vi "Machine.vi"   [LabVIEW 2011]
doc: "使用该模板构建标准状态机设计模式。各状态执行代码并决定转移状态。将该设计模式与根据用户动作响应而执行代码的用户界面事件处理器模式相比较。同时将该设计模式与队列消息处理模式（各消息处理代码可排队0个或多个新消息）。"
uses:
  MachineState.ctl
  F1State.ctl
  API/API DYM.lvlib
types:
  T1 = typedef "MachineState.ctl" = enum16{"Initialize", "一号平台分拣运输", "二号平台运输物料", "三号平台气动机械手运输物料", "三号平台运输机构运输物料", "Stop"}
  T2 = typedef "F1State.ctl" = enum16{"Initialize", "Stop", "推送物料", "推料气缸复位", "物件到位检测-光电漫射", "物体属性检测-电涡流", "分拣物体", "不分拣物体", "物件到位检测-电容式接近开关", "气缸机构运动", "气缸机构复位"}
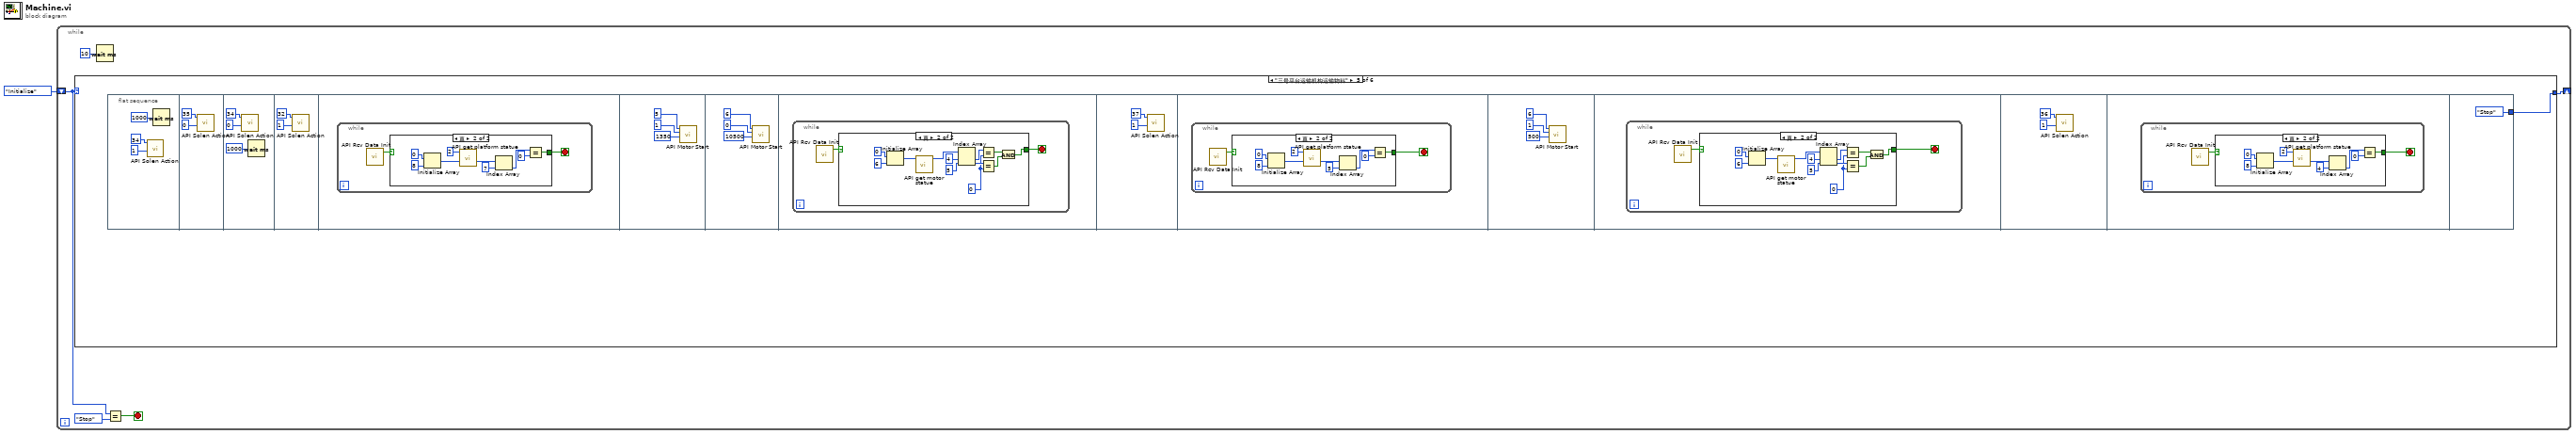
[diagram p0: block diagram]
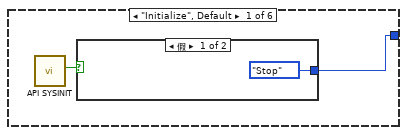
[diagram p2: hidden frame]
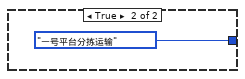
[diagram p3: hidden frame]
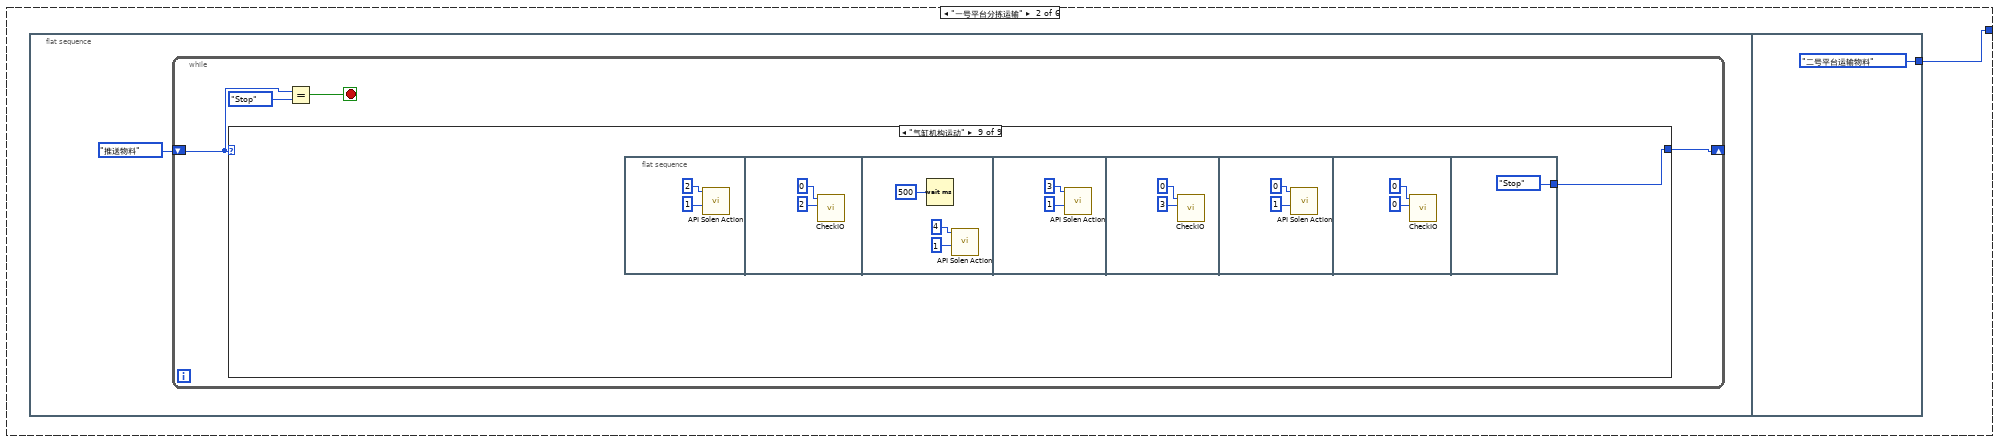
[diagram p4: hidden frame]
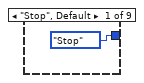
[diagram p5: hidden frame]
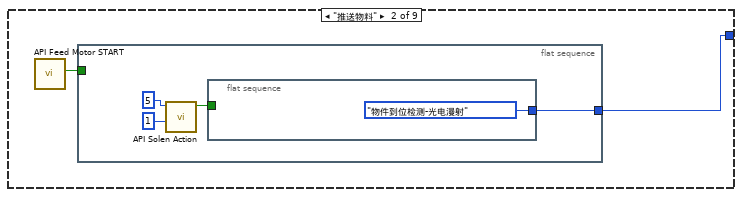
[diagram p6: hidden frame]
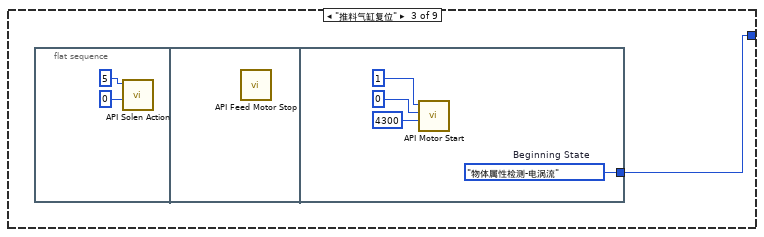
[diagram p7: hidden frame]
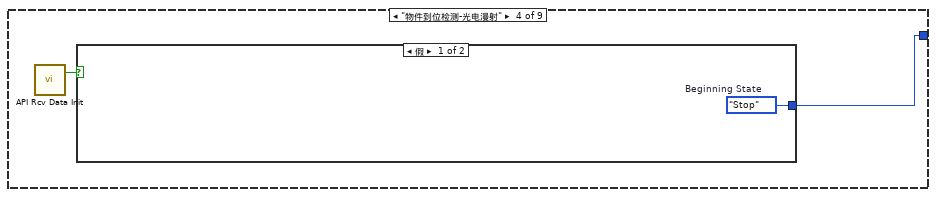
[diagram p8: hidden frame]
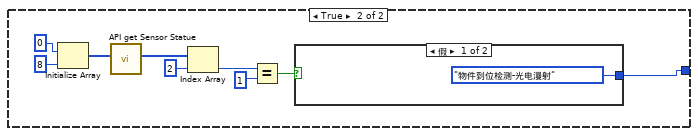
[diagram p9: hidden frame]
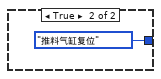
[diagram p10: hidden frame]
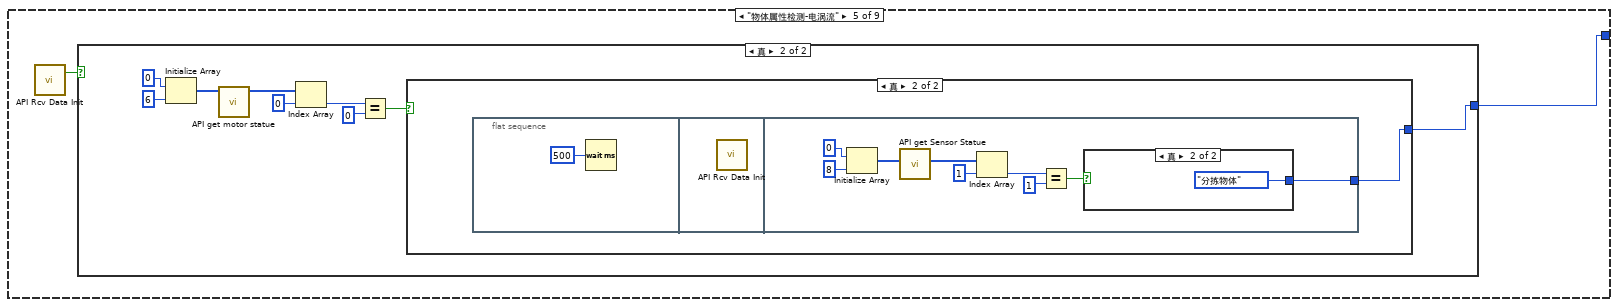
[diagram p11: hidden frame]
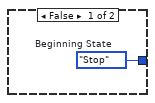
[diagram p12: hidden frame]
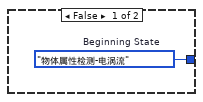
[diagram p13: hidden frame]
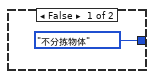
[diagram p14: hidden frame]
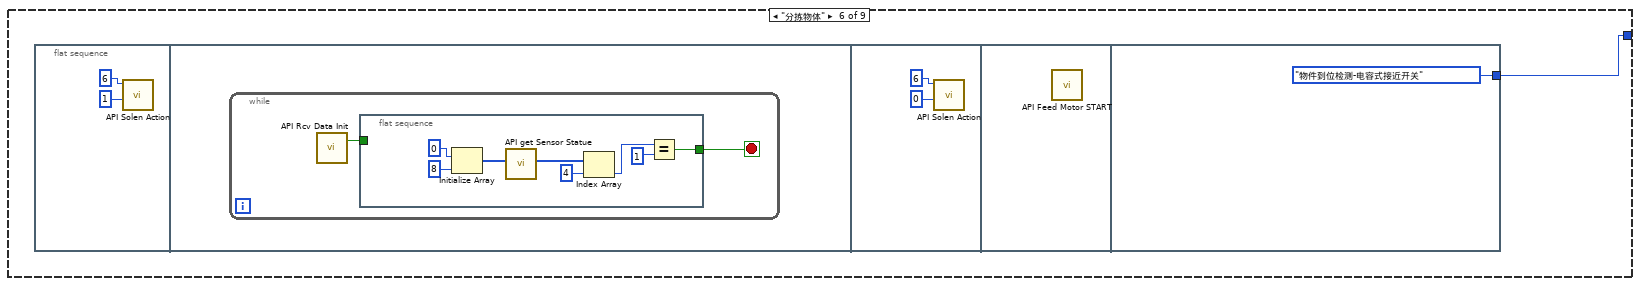
[diagram p15: hidden frame]
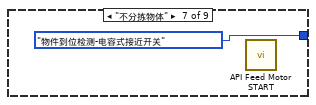
[diagram p16: hidden frame]
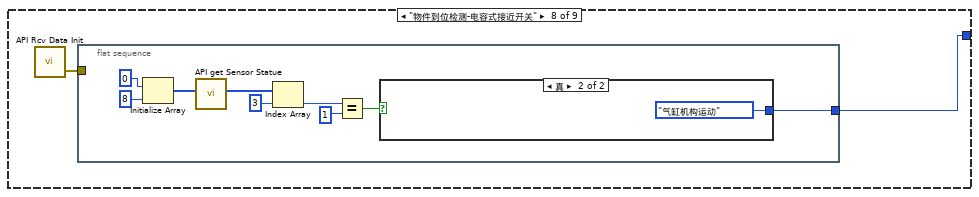
[diagram p17: hidden frame]
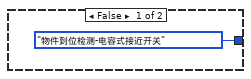
[diagram p18: hidden frame]
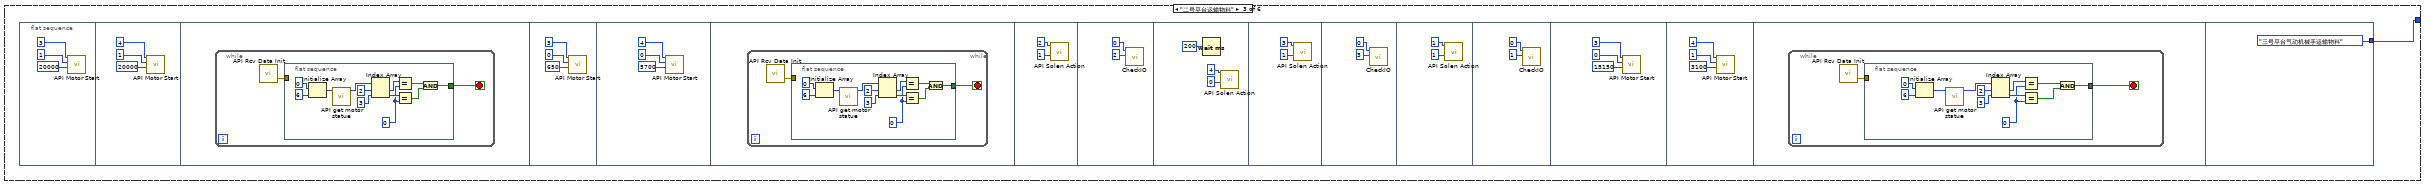
[diagram p19: hidden frame]
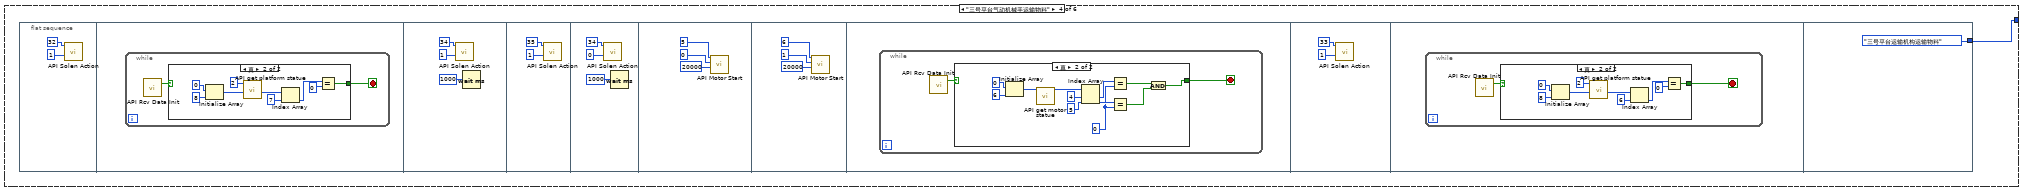
[diagram p20: hidden frame]
diagram:
  n1 = while {
    shift-right: [w2] -> _
    shift-left: MachineState."Initialize" ("Beginning State") -> [w4]
    stop <- w6 stop-if-true
    n2 = case shown="\"三号平台运输机构运输物料\"" w4 {
      tunnel: [w7 w11 w120 w197 w256 MachineState."Stop" ("Beginning State")] -> w2
      frame "Initialize", Default {
        n3 = call "API SYSINIT.vi"() -> ("SYSINIT return value"=w8:bool)  [unwired: 11 in]
        n4 = case shown="假" w8 {
          tunnel: [MachineState."Stop" ("Beginning State") MachineState."一号平台分拣运输" ("Beginning State")] -> w7
          frame False {
          }
          frame True {
          }
        }
      }
      frame "一号平台分拣运输" {
        n5 = flat-sequence {
          tunnel: [MachineState."二号平台运输物料" ("Beginning State")] -> w11
          frame #0 {
            n6 = while {
              shift-right: [w13] -> _
              shift-left: F1State."推送物料" ("Beginning State") -> [w14]
              stop <- w16 stop-if-true
              n7 = case shown="\"气缸机构运动\"" w14 {
                tunnel: [F1State."Stop" ("Beginning State") w19 w25 w32 w46 w72 F1State."物件到位检测-电容式接近开关" ("Beginning State") w89 w102] -> w13
                frame "Stop", Default {
                }
                frame "推送物料" {
                  n8 = call "API Feed Motor START.vi"() -> ("feedmotorstart return value"=w18:bool)  [unwired: 11 in]
                  n9 = flat-sequence {
                    tunnel: [w20] -> w19
                    tunnel: w18 -> [_]
                    frame #0 {
                      n10 = call "API Solen Action.vi"("statue"=1, "solenNum"=5) -> ("solenaction return value"=w21:bool)  [unwired: 9 in]
                      n11 = flat-sequence {
                        tunnel: w21 -> [_]
                        tunnel: [F1State."物件到位检测-光电漫射" ("Beginning State")] -> w20
                        frame #0 {
                        }
                      }
                    }
                  }
                }
                frame "推料气缸复位" {
                  n12 = flat-sequence {
                    tunnel: [w28] -> w25
                    frame #0 {
                      n13 = call "API Solen Action.vi"("statue"=0, "solenNum"=5) -> ()  [unwired: 9 in, 1 out]
                    }
                    frame #1 {
                      n14 = call "API Feed Motor Stop.vi"() -> ()  [unwired: 11 in, 1 out]
                    }
                    frame #2 {
                      w28 = F1State."物体属性检测-电涡流"  # Beginning State
                      n15 = call "API Motor Start.vi"("stepNum"=4300, "direction"=0, "motorNum"=1) -> ()  [unwired: 8 in, 1 out]
                    }
                  }
                }
                frame "物件到位检测-光电漫射" {
                  n16 = call "API Rcv Data Init.vi"() -> ("RTV"=w33:bool)  [unwired: 2 in, 1 out]
                  n17 = case shown="假" w33 {
                    tunnel: [w34 w35] -> w32
                    frame False {
                      w34 = F1State."Stop"  # Beginning State
                    }
                    frame True {
                      n18 = Initialize Array(0 ("元素"), 8 ("维数大小")) -> (w41:i32[])
                      n19 = call "API get Sensor Statue.vi"("array input"=w41) -> ("array output"=w40:i32[])  [unwired: 9 in, 1 out]
                      n20 = Index Array(array=w40, index=2 ("索引")) -> (element=w38:i32)
                      n21 = Equal?(x=w38, y=1) -> (x = y?=w36:bool)
                      n22 = case shown="假" w36 {
                        tunnel: [F1State."物件到位检测-光电漫射" ("Beginning State") F1State."推料气缸复位" ("Beginning State")] -> w35
                        frame False {
                        }
                        frame True {
                        }
                      }
                    }
                  }
                }
                frame "物体属性检测-电涡流" {
                  n23 = call "API Rcv Data Init.vi"() -> ("RTV"=w47:bool)  [unwired: 2 in, 1 out]
                  n24 = case shown="真" w47 {
                    tunnel: [w48 w49] -> w46
                    frame False {
                      w48 = F1State."Stop"  # Beginning State
                    }
                    frame True {
                      n25 = Initialize Array(0 ("元素"), 6 ("维数大小")) -> (w55:i32[])
                      n26 = call "API get motor statue.vi"("motor statue array input"=w55) -> ("motor statue array output"=w54:i32[])  [unwired: 9 in, 1 out]
                      n27 = Index Array(array=w54, index=0 ("索引")) -> (element=w52:i32)
                      n28 = Equal?(x=w52, y=0) -> (x = y?=w50:bool)
                      n29 = case shown="真" w50 {
                        tunnel: [w58 w59] -> w49
                        frame False {
                          w58 = F1State."物体属性检测-电涡流"  # Beginning State
                        }
                        frame True {
                          n30 = flat-sequence {
                            tunnel: [w61] -> w59
                            frame #0 {
                              n31 = Wait (ms)(milliseconds to wait=u32 500) -> ()  [unwired: 1 out]
                            }
                            frame #1 {
                              n32 = call "API Rcv Data Init.vi"() -> ()  [unwired: 2 in, 2 out]
                            }
                            frame #2 {
                              n33 = Initialize Array(0 ("元素"), 8 ("维数大小")) -> (w67:i32[])
                              n34 = call "API get Sensor Statue.vi"("array input"=w67) -> ("array output"=w66:i32[])  [unwired: 9 in, 1 out]
                              n35 = Index Array(array=w66, index=1 ("索引")) -> (element=w63:i32)
                              n36 = Equal?(x=w63, y=1) -> (x = y?=w62:bool)
                              n37 = case shown="真" w62 {
                                tunnel: [F1State."不分拣物体" ("Beginning State") F1State."分拣物体" ("Beginning State")] -> w61
                                frame False {
                                }
                                frame True {
                                }
                              }
                            }
                          }
                        }
                      }
                    }
                  }
                }
                frame "分拣物体" {
                  n38 = flat-sequence {
                    tunnel: [F1State."物件到位检测-电容式接近开关" ("Beginning State")] -> w72
                    frame #0 {
                      n39 = call "API Solen Action.vi"("statue"=1, "solenNum"=6) -> ()  [unwired: 9 in, 1 out]
                    }
                    frame #1 {
                      n40 = while {
                        stop <- w76 stop-if-true
                        n41 = call "API Rcv Data Init.vi"() -> ("RTV"=w75:bool)  [unwired: 2 in, 1 out]
                        n42 = flat-sequence {
                          tunnel: [w77] -> w76
                          tunnel: w75 -> [_]
                          frame #0 {
                            n43 = Initialize Array(0 ("元素"), 8 ("维数大小")) -> (w82:i32[])
                            n44 = call "API get Sensor Statue.vi"("array input"=w82) -> ("array output"=w81:i32[])  [unwired: 9 in, 1 out]
                            n45 = Index Array(array=w81, index=4 ("索引")) -> (element=w79:i32)
                            n46 = Equal?(x=w79, y=1) -> (x = y?=w77:bool)
                          }
                        }
                      }
                    }
                    frame #2 {
                      n47 = call "API Solen Action.vi"("statue"=0, "solenNum"=6) -> ()  [unwired: 9 in, 1 out]
                    }
                    frame #3 {
                      n48 = call "API Feed Motor START.vi"() -> ()  [unwired: 11 in, 1 out]
                    }
                    frame #4 {
                    }
                  }
                }
                frame "不分拣物体" {
                  n49 = call "API Feed Motor START.vi"() -> ()  [unwired: 11 in, 1 out]
                }
                frame "物件到位检测-电容式接近开关" {
                  n50 = call "API Rcv Data Init.vi"() -> ("错误输出"=w90:errorcluster)  [unwired: 2 in, 1 out]
                  n51 = flat-sequence {
                    tunnel: w90 -> [_]
                    tunnel: [w91] -> w89
                    frame #0 {
                      n52 = Initialize Array(0 ("元素"), 8 ("维数大小")) -> (w97:i32[])
                      n53 = call "API get Sensor Statue.vi"("array input"=w97) -> ("array output"=w96:i32[])  [unwired: 9 in, 1 out]
                      n54 = Index Array(array=w96, index=3 ("索引")) -> (element=w94:i32)
                      n55 = Equal?(x=w94, y=1) -> (x = y?=w92:bool)
                      n56 = case shown="真" w92 {
                        tunnel: [F1State."物件到位检测-电容式接近开关" ("Beginning State") F1State."气缸机构运动" ("Beginning State")] -> w91
                        frame False {
                        }
                        frame True {
                        }
                      }
                    }
                  }
                }
                frame "气缸机构运动" {
                  n57 = flat-sequence {
                    tunnel: [F1State."Stop" ("Beginning State")] -> w102
                    frame #0 {
                      n58 = call "API Solen Action.vi"("statue"=1, "solenNum"=2) -> ()  [unwired: 9 in, 1 out]
                    }
                    frame #1 {
                      n59 = call "CheckIO.vi"("IONum"=2, "PlatformNum"=0) -> ()  [unwired: 10 in]
                    }
                    frame #2 {
                      n60 = Wait (ms)(milliseconds to wait=u32 500) -> ()  [unwired: 1 out]
                      n61 = call "API Solen Action.vi"("statue"=1, "solenNum"=4) -> ()  [unwired: 9 in, 1 out]
                    }
                    frame #3 {
                      n62 = call "API Solen Action.vi"("statue"=1, "solenNum"=3) -> ()  [unwired: 9 in, 1 out]
                    }
                    frame #4 {
                      n63 = call "CheckIO.vi"("IONum"=3, "PlatformNum"=0) -> ()  [unwired: 10 in]
                    }
                    frame #5 {
                      n64 = call "API Solen Action.vi"("statue"=1, "solenNum"=0) -> ()  [unwired: 9 in, 1 out]
                    }
                    frame #6 {
                      n65 = call "CheckIO.vi"("IONum"=0, "PlatformNum"=0) -> ()  [unwired: 10 in]
                    }
                    frame #7 {
                    }
                  }
                }
              }
              n66 = Equal?(x=w14, y=F1State."Stop" ("Beginning State")) -> (x = y?=w16:bool)
            }
          }
          frame #1 {
          }
        }
      }
      frame "二号平台运输物料" {
        n67 = flat-sequence {
          tunnel: [MachineState."三号平台气动机械手运输物料" ("Beginning State")] -> w120
          frame #0 {
            n68 = call "API Motor Start.vi"("stepNum"=20000, "direction"=1, "motorNum"=3) -> ()  [unwired: 8 in, 1 out]
          }
          frame #1 {
            n69 = call "API Motor Start.vi"("stepNum"=20000, "direction"=1, "motorNum"=4) -> ()  [unwired: 8 in, 1 out]
          }
          frame #2 {
            n70 = while {
              stop <- w127 stop-if-true
              n71 = call "API Rcv Data Init.vi"() -> ("错误输出"=w128:errorcluster)  [unwired: 2 in, 1 out]
              n72 = flat-sequence {
                tunnel: w128 -> [_]
                tunnel: [w129] -> w127
                frame #0 {
                  w132 = 0
                  n73 = Initialize Array(0 ("元素"), 6 ("维数大小")) -> (w138:i32[])
                  n74 = call "API get motor statue.vi"("motor statue array input"=w138) -> ("motor statue array output"=w137:i32[])  [unwired: 9 in, 1 out]
                  n75 = Index Array(array=w137, index #1=2 ("索引"), index #2=3 ("索引")) -> (element #1=w134:i32, element #2=w133:i32)
                  n76 = Equal?(x=w134, y=w132) -> (x = y?=w131:bool)
                  n77 = Equal?(x=w133, y=w132) -> (x = y?=w130:bool)
                  n78 = And(x=w131, y=w130) -> (x .and. y?=w129:bool)
                }
              }
            }
          }
          frame #3 {
            n79 = call "API Motor Start.vi"("stepNum"=650, "direction"=0, "motorNum"=3) -> ()  [unwired: 8 in, 1 out]
          }
          frame #4 {
            n80 = call "API Motor Start.vi"("stepNum"=5700, "direction"=0, "motorNum"=4) -> ()  [unwired: 8 in, 1 out]
          }
          frame #5 {
            n81 = while {
              stop <- w147 stop-if-true
              n82 = call "API Rcv Data Init.vi"() -> ("错误输出"=w148:errorcluster)  [unwired: 2 in, 1 out]
              n83 = flat-sequence {
                tunnel: w148 -> [_]
                tunnel: [w149] -> w147
                frame #0 {
                  w152 = 0
                  n84 = Initialize Array(0 ("元素"), 6 ("维数大小")) -> (w158:i32[])
                  n85 = call "API get motor statue.vi"("motor statue array input"=w158) -> ("motor statue array output"=w157:i32[])  [unwired: 9 in, 1 out]
                  n86 = Index Array(array=w157, index #1=2 ("索引"), index #2=3 ("索引")) -> (element #1=w154:i32, element #2=w153:i32)
                  n87 = Equal?(x=w154, y=w152) -> (x = y?=w151:bool)
                  n88 = Equal?(x=w153, y=w152) -> (x = y?=w150:bool)
                  n89 = And(x=w151, y=w150) -> (x .and. y?=w149:bool)
                }
              }
            }
          }
          frame #6 {
            n90 = call "API Solen Action.vi"("statue"=1, "solenNum"=2) -> ()  [unwired: 9 in, 1 out]
          }
          frame #7 {
            n91 = call "CheckIO.vi"("IONum"=2, "PlatformNum"=0) -> ()  [unwired: 10 in]
          }
          frame #8 {
            n92 = Wait (ms)(milliseconds to wait=u32 200 ("等待时间（毫秒）")) -> ()  [unwired: 1 out]
            n93 = call "API Solen Action.vi"("statue"=0, "solenNum"=4) -> ()  [unwired: 9 in, 1 out]
          }
          frame #9 {
            n94 = call "API Solen Action.vi"("statue"=1, "solenNum"=3) -> ()  [unwired: 9 in, 1 out]
          }
          frame #10 {
            n95 = call "CheckIO.vi"("IONum"=3, "PlatformNum"=0) -> ()  [unwired: 10 in]
          }
          frame #11 {
            n96 = call "API Solen Action.vi"("statue"=1, "solenNum"=1) -> ()  [unwired: 9 in, 1 out]
          }
          frame #12 {
            n97 = call "CheckIO.vi"("IONum"=1, "PlatformNum"=0) -> ()  [unwired: 10 in]
          }
          frame #13 {
            n98 = call "API Motor Start.vi"("stepNum"=15150, "direction"=0, "motorNum"=3) -> ()  [unwired: 8 in, 1 out]
          }
          frame #14 {
            n99 = call "API Motor Start.vi"("stepNum"=3100, "direction"=1, "motorNum"=4) -> ()  [unwired: 8 in, 1 out]
          }
          frame #15 {
            n100 = while {
              stop <- w182 stop-if-true
              n101 = call "API Rcv Data Init.vi"() -> ("错误输出"=w183:errorcluster)  [unwired: 2 in, 1 out]
              n102 = flat-sequence {
                tunnel: w183 -> [_]
                tunnel: [w184] -> w182
                frame #0 {
                  w187 = 0
                  n103 = Initialize Array(0 ("元素"), 6 ("维数大小")) -> (w193:i32[])
                  n104 = call "API get motor statue.vi"("motor statue array input"=w193) -> ("motor statue array output"=w192:i32[])  [unwired: 9 in, 1 out]
                  n105 = Index Array(array=w192, index #1=2 ("索引"), index #2=3 ("索引")) -> (element #1=w189:i32, element #2=w188:i32)
                  n106 = Equal?(x=w189, y=w187) -> (x = y?=w186:bool)
                  n107 = Equal?(x=w188, y=w187) -> (x = y?=w185:bool)
                  n108 = And(x=w186, y=w185) -> (x .and. y?=w184:bool)
                }
              }
            }
          }
          frame #16 {
          }
        }
      }
      frame "三号平台气动机械手运输物料" {
        n109 = flat-sequence {
          tunnel: [MachineState."三号平台运输机构运输物料" ("Beginning State")] -> w197
          frame #0 {
            n110 = call "API Solen Action.vi"("statue"=1, "solenNum"=32) -> ()  [unwired: 9 in, 1 out]
          }
          frame #1 {
            n111 = while {
              stop <- w200 stop-if-true
              n112 = call "API Rcv Data Init.vi"() -> ("RTV"=w201:bool)  [unwired: 2 in, 1 out]
              n113 = case shown="真" w201 {
                selector: w201 -> [w202 _]
                tunnel: [w202 w203] -> w200
                frame False {
                }
                frame True {
                  n114 = Initialize Array(0 ("元素"), 8 ("维数大小")) -> (w208:i32[])
                  n115 = call "API get platform statue.vi"("platformStatue input"=w208, "PlatformNum"=2) -> ("platformStatue output"=w207:i32[])  [unwired: 8 in, 1 out]
                  n116 = Index Array(array=w207, index=7 ("索引")) -> (element=w205:i32)
                  n117 = Equal?(x=w205, y=0) -> (x = y?=w203:bool)
                }
              }
            }
          }
          frame #2 {
            n118 = call "API Solen Action.vi"("statue"=1, "solenNum"=34) -> ()  [unwired: 9 in, 1 out]
            n119 = Wait (ms)(milliseconds to wait=u32 1000 ("等待时间（毫秒）")) -> ()  [unwired: 1 out]
          }
          frame #3 {
            n120 = call "API Solen Action.vi"("statue"=1, "solenNum"=35) -> ()  [unwired: 9 in, 1 out]
          }
          frame #4 {
            n121 = call "API Solen Action.vi"("statue"=0, "solenNum"=34) -> ()  [unwired: 9 in, 1 out]
            n122 = Wait (ms)(milliseconds to wait=u32 1000 ("等待时间（毫秒）")) -> ()  [unwired: 1 out]
          }
          frame #5 {
            n123 = call "API Motor Start.vi"("stepNum"=20000, "direction"=0, "motorNum"=5) -> ()  [unwired: 8 in, 1 out]
          }
          frame #6 {
            n124 = call "API Motor Start.vi"("stepNum"=20000, "direction"=1, "motorNum"=6) -> ()  [unwired: 8 in, 1 out]
          }
          frame #7 {
            n125 = while {
              stop <- w226 stop-if-true
              n126 = call "API Rcv Data Init.vi"() -> ("RTV"=w227:bool)  [unwired: 2 in, 1 out]
              n127 = case shown="真" w227 {
                selector: w227 -> [w228 _]
                tunnel: [w228 w229] -> w226
                frame False {
                }
                frame True {
                  w232 = 0
                  n128 = Initialize Array(0 ("元素"), 6 ("维数大小")) -> (w237:i32[])
                  n129 = call "API get motor statue.vi"("motor statue array input"=w237) -> ("motor statue array output"=w236:i32[])  [unwired: 9 in, 1 out]
                  n130 = Index Array(array=w236, index #1=4 ("索引"), index #2=5 ("索引")) -> (element #1=w234:i32, element #2=w233:i32)
                  n131 = Equal?(x=w234, y=w232) -> (x = y?=w231:bool)
                  n132 = Equal?(x=w233, y=w232) -> (x = y?=w230:bool)
                  n133 = And(x=w231, y=w230) -> (x .and. y?=w229:bool)
                }
              }
            }
          }
          frame #8 {
            n134 = call "API Solen Action.vi"("statue"=1, "solenNum"=33) -> ()  [unwired: 9 in, 1 out]
          }
          frame #9 {
            n135 = while {
              stop <- w243 stop-if-true
              n136 = call "API Rcv Data Init.vi"() -> ("RTV"=w244:bool)  [unwired: 2 in, 1 out]
              n137 = case shown="真" w244 {
                selector: w244 -> [w245 _]
                tunnel: [w245 w246] -> w243
                frame False {
                }
                frame True {
                  n138 = Initialize Array(0 ("元素"), 8 ("维数大小")) -> (w251:i32[])
                  n139 = call "API get platform statue.vi"("platformStatue input"=w251, "PlatformNum"=2) -> ("platformStatue output"=w250:i32[])  [unwired: 8 in, 1 out]
                  n140 = Index Array(array=w250, index=6 ("索引")) -> (element=w248:i32)
                  n141 = Equal?(x=w248, y=0) -> (x = y?=w246:bool)
                }
              }
            }
          }
          frame #10 {
          }
        }
      }
      frame "三号平台运输机构运输物料" {
        n142 = flat-sequence {
          tunnel: [MachineState."Stop" ("Beginning State")] -> w256
          frame #0 {
            n143 = call "API Solen Action.vi"("statue"=1, "solenNum"=34) -> ()  [unwired: 9 in, 1 out]
            n144 = Wait (ms)(milliseconds to wait=u32 1000 ("等待时间（毫秒）")) -> ()  [unwired: 1 out]
          }
          frame #1 {
            n145 = call "API Solen Action.vi"("statue"=0, "solenNum"=35) -> ()  [unwired: 9 in, 1 out]
          }
          frame #2 {
            n146 = call "API Solen Action.vi"("statue"=0, "solenNum"=34) -> ()  [unwired: 9 in, 1 out]
            n147 = Wait (ms)(milliseconds to wait=u32 1000 ("等待时间（毫秒）")) -> ()  [unwired: 1 out]
          }
          frame #3 {
            n148 = call "API Solen Action.vi"("statue"=1, "solenNum"=32) -> ()  [unwired: 9 in, 1 out]
          }
          frame #4 {
            n149 = while {
              stop <- w267 stop-if-true
              n150 = call "API Rcv Data Init.vi"() -> ("RTV"=w268:bool)  [unwired: 2 in, 1 out]
              n151 = case shown="真" w268 {
                selector: w268 -> [w269 _]
                tunnel: [w269 w270] -> w267
                frame False {
                }
                frame True {
                  n152 = Initialize Array(0 ("元素"), 8 ("维数大小")) -> (w275:i32[])
                  n153 = call "API get platform statue.vi"("platformStatue input"=w275, "PlatformNum"=2) -> ("platformStatue output"=w274:i32[])  [unwired: 8 in, 1 out]
                  n154 = Index Array(array=w274, index=7 ("索引")) -> (element=w272:i32)
                  n155 = Equal?(x=w272, y=0) -> (x = y?=w270:bool)
                }
              }
            }
          }
          frame #5 {
            n156 = call "API Motor Start.vi"("stepNum"=1350, "direction"=1, "motorNum"=5) -> ()  [unwired: 8 in, 1 out]
          }
          frame #6 {
            n157 = call "API Motor Start.vi"("stepNum"=10500, "direction"=0, "motorNum"=6) -> ()  [unwired: 8 in, 1 out]
          }
          frame #7 {
            n158 = while {
              stop <- w285 stop-if-true
              n159 = call "API Rcv Data Init.vi"() -> ("RTV"=w286:bool)  [unwired: 2 in, 1 out]
              n160 = case shown="真" w286 {
                selector: w286 -> [w287 _]
                tunnel: [w287 w288] -> w285
                frame False {
                }
                frame True {
                  w291 = 0
                  n161 = Initialize Array(0 ("元素"), 6 ("维数大小")) -> (w296:i32[])
                  n162 = call "API get motor statue.vi"("motor statue array input"=w296) -> ("motor statue array output"=w295:i32[])  [unwired: 9 in, 1 out]
                  n163 = Index Array(array=w295, index #1=4 ("索引"), index #2=5 ("索引")) -> (element #1=w293:i32, element #2=w292:i32)
                  n164 = Equal?(x=w293, y=w291) -> (x = y?=w290:bool)
                  n165 = Equal?(x=w292, y=w291) -> (x = y?=w289:bool)
                  n166 = And(x=w290, y=w289) -> (x .and. y?=w288:bool)
                }
              }
            }
          }
          frame #8 {
            n167 = call "API Solen Action.vi"("statue"=1, "solenNum"=37) -> ()  [unwired: 9 in, 1 out]
          }
          frame #9 {
            n168 = while {
              stop <- w302 stop-if-true
              n169 = call "API Rcv Data Init.vi"() -> ("RTV"=w303:bool)  [unwired: 2 in, 1 out]
              n170 = case shown="真" w303 {
                selector: w303 -> [w304 _]
                tunnel: [w304 w305] -> w302
                frame False {
                }
                frame True {
                  n171 = Initialize Array(0 ("元素"), 8 ("维数大小")) -> (w310:i32[])
                  n172 = call "API get platform statue.vi"("platformStatue input"=w310, "PlatformNum"=2) -> ("platformStatue output"=w309:i32[])  [unwired: 8 in, 1 out]
                  n173 = Index Array(array=w309, index=5 ("索引")) -> (element=w307:i32)
                  n174 = Equal?(x=w307, y=0) -> (x = y?=w305:bool)
                }
              }
            }
          }
          frame #10 {
            n175 = call "API Motor Start.vi"("stepNum"=500, "direction"=1, "motorNum"=6) -> ()  [unwired: 8 in, 1 out]
          }
          frame #11 {
            n176 = while {
              stop <- w317 stop-if-true
              n177 = call "API Rcv Data Init.vi"() -> ("RTV"=w318:bool)  [unwired: 2 in, 1 out]
              n178 = case shown="真" w318 {
                selector: w318 -> [w319 _]
                tunnel: [w319 w320] -> w317
                frame False {
                }
                frame True {
                  w323 = 0
                  n179 = Initialize Array(0 ("元素"), 6 ("维数大小")) -> (w328:i32[])
                  n180 = call "API get motor statue.vi"("motor statue array input"=w328) -> ("motor statue array output"=w327:i32[])  [unwired: 9 in, 1 out]
                  n181 = Index Array(array=w327, index #1=4 ("索引"), index #2=5 ("索引")) -> (element #1=w325:i32, element #2=w324:i32)
                  n182 = Equal?(x=w325, y=w323) -> (x = y?=w322:bool)
                  n183 = Equal?(x=w324, y=w323) -> (x = y?=w321:bool)
                  n184 = And(x=w322, y=w321) -> (x .and. y?=w320:bool)
                }
              }
            }
          }
          frame #12 {
            n185 = call "API Solen Action.vi"("statue"=1, "solenNum"=36) -> ()  [unwired: 9 in, 1 out]
          }
          frame #13 {
            n186 = while {
              stop <- w334 stop-if-true
              n187 = call "API Rcv Data Init.vi"() -> ("RTV"=w335:bool)  [unwired: 2 in, 1 out]
              n188 = case shown="真" w335 {
                selector: w335 -> [w336 _]
                tunnel: [w336 w337] -> w334
                frame False {
                }
                frame True {
                  n189 = Initialize Array(0 ("元素"), 8 ("维数大小")) -> (w342:i32[])
                  n190 = call "API get platform statue.vi"("platformStatue input"=w342, "PlatformNum"=2) -> ("platformStatue output"=w341:i32[])  [unwired: 8 in, 1 out]
                  n191 = Index Array(array=w341, index=4 ("索引")) -> (element=w339:i32)
                  n192 = Equal?(x=w339, y=0) -> (x = y?=w337:bool)
                }
              }
            }
          }
          frame #14 {
          }
        }
      }
      frame "Stop" {
        n193 = call "API SYSQUIT.vi"() -> ()  [unwired: 12 in]
      }
    }
    n194 = Wait (ms)(milliseconds to wait=u32 10) -> ()  [unwired: 1 out]
    n195 = Equal?(x=w4, y=MachineState."Stop" ("States")) -> (x = y?=w6:bool)
  }
